vi "readBin(U32).vi"(9 "Size":i32, 10 "Offset":i32, 11 "Buffer IN":string) -> (1 "Int (U32)":u32, 2 "Offset+Size":i32, 3 "Buffer OUT":string)   [LabVIEW 2017, in "HEKAdat.lvclass"]
uses:
  HEKAdat.lvclass
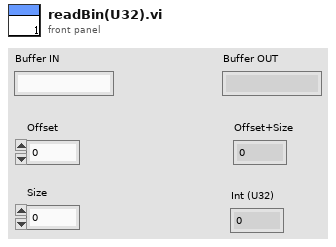
[diagram p1: front panel]
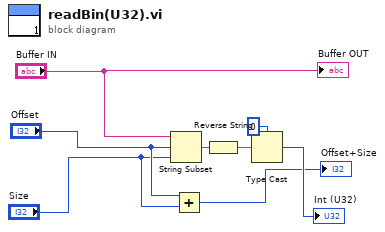
[diagram p0: block diagram]
diagram:
  n1 = String Subset(string="Buffer IN", offset (0)="Offset", length (rest)="Size") -> (substring=w5:string)
  n2 = Add(x="Offset", y="Size") -> (x+y=→"Offset+Size":i32)
  n3 = Reverse String(1:w5) -> (0:w6:string)
  n4 = Type Cast(type=u32 0, x=w6) -> (*(type *) &x=→"Int (U32)":u32)
  "Buffer OUT" <- "Buffer IN"
